vi "locked.vi"() -> ()   [LabVIEW 2020]
panel:
  out "Locked":bool
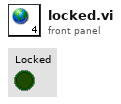
[diagram p1: front panel]
diagram:
